vi "Activity Log Write Log and Rollover.vi"(8 "error in (no error)":errorcluster, 9 "Max Size":i32=100000, 10 "Log Text":string, 11 "Log File":path) -> (0 "error out":errorcluster, 2 "new file?":bool, 3 "Log File out":path)   [LabVIEW 2021]
doc: "Post-Certification Software"
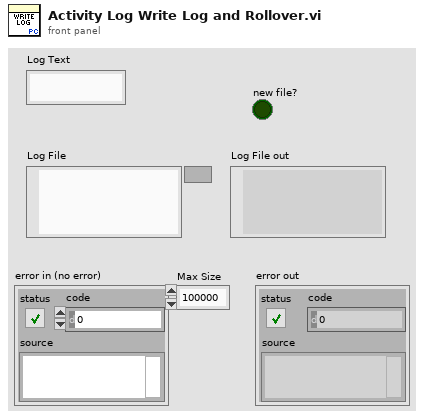
[diagram p1: front panel]
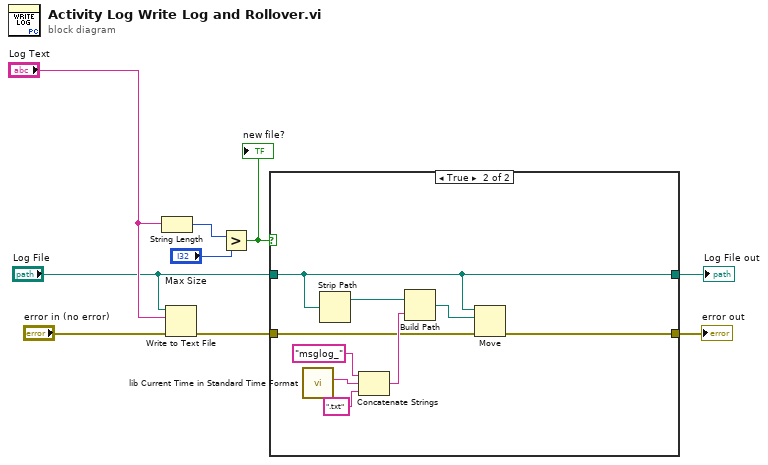
[diagram p0: block diagram]
diagram:
  n1 = String Length(string="Log Text") -> (length=w7:i32)
  n2 = Write to Text File(file (use dialog)="Log File", text="Log Text", error in="error in (no error)") -> (error out=w4:errorcluster)  [unwired: 1 in, 2 out]
  n3 = Greater?(x=w7, y="Max Size") -> (0:w5:bool)
  "new file?" <- w5
  n4 = case shown="True" w5 {
    tunnel: w4 -> [w11 w15]
    tunnel: [w11 w13] -> w3
    tunnel: "Log File" -> [w10 w12]
    tunnel: [w10 w12] -> w1
    frame False {
    }
    frame True {
      n5 = call "lib Current Time in Standard Time Format.vi"() -> ("date/time string"=w20:string)  [unwired: 11 in]
      n6 = Strip Path(path=w12) -> (stripped path=w16:path)  [unwired: 1 out]
      n7 = Concatenate Strings("msglog_" ("string"), w20, ".txt" ("string")) -> (w17:string)
      n8 = Build Path(base path=w16, name or relative path=w17) -> (appended path=w14:path)
      n9 = Move(source path=w12, error in=w15, 10:w14) -> (error out=w13:errorcluster)  [unwired: 2 in, 2 out]
    }
  }
  "error out" <- w3
  "Log File out" <- w1
